vi "configureOutput.vi"(6 "sofwareTrigger?":bool, 8 "error in (no error)":errorcluster, 9 "Data":variant, 10 "Config":T1, 11 "SpinCore in":refnum<class "SpinCore.lvclass">) -> (0 "error out":errorcluster, 3 "SpinCore out":refnum<class "SpinCore.lvclass">)   [LabVIEW 2009, in "Hardware.lvlib" / "Channels.lvlib" / "SpinCore.lvclass"]
doc: "Data is a varient cluster. \n\nThe varient is transformed into the correct cluster, and that cluster is stored.\n(Not Implemented for Ramp function)"
uses:
  SpinCore.lvclass
  Generic/DDSOutput.lvclass
  SpinCore.lvclass/SpinCore.ctl
panel:
  out "Data":dbl
  out "load time":dbl
  out "data (time, freq, amplitude, phase)":dbl[][](array[numeric]) format="%#.7g"
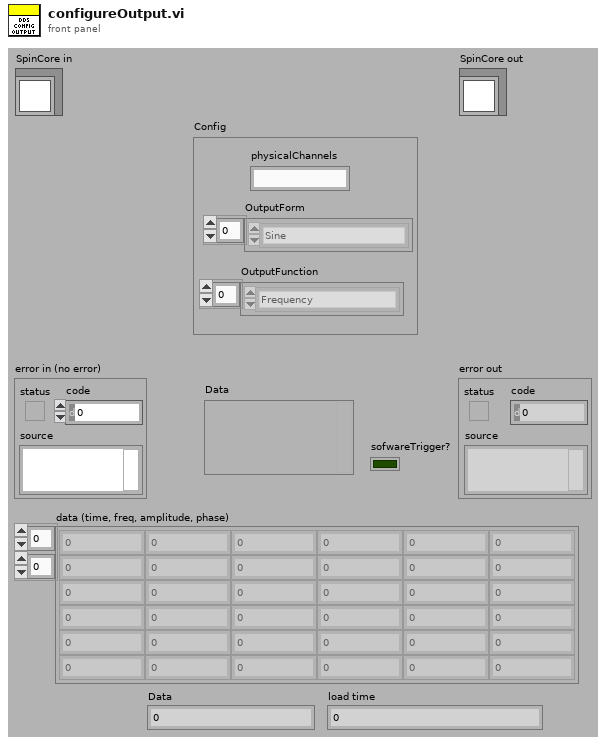
[diagram p1: front panel]
types:
  T1 = cluster{"OutputForm":enum16{"Sine", "Square", "Triangle", "Arbitrary"}[], "OutputFunction":enum16{"Frequency", "Ramp", "Sequence"}[], "physicalChannels":string}
  T2 = cluster{"Frequency(MHz)":dbl, "Amplitude":dbl, "Phase":dbl, "OutputForm":enum16{"Sine", "Square", "Triangle", "Arbitrary"}}[]
  T3 = cluster{"data (time, freq, amplitude, phase)":dbl[][]}
  T4 = cluster{"data (time, freq, amplitude, phase)":dbl[][]}[]
  T5 = cluster{"Frequency(MHz)":dbl, "Amplitude":dbl, "Phase":dbl, "OutputForm":enum16{"Sine", "Square", "Triangle", "Arbitrary"}}
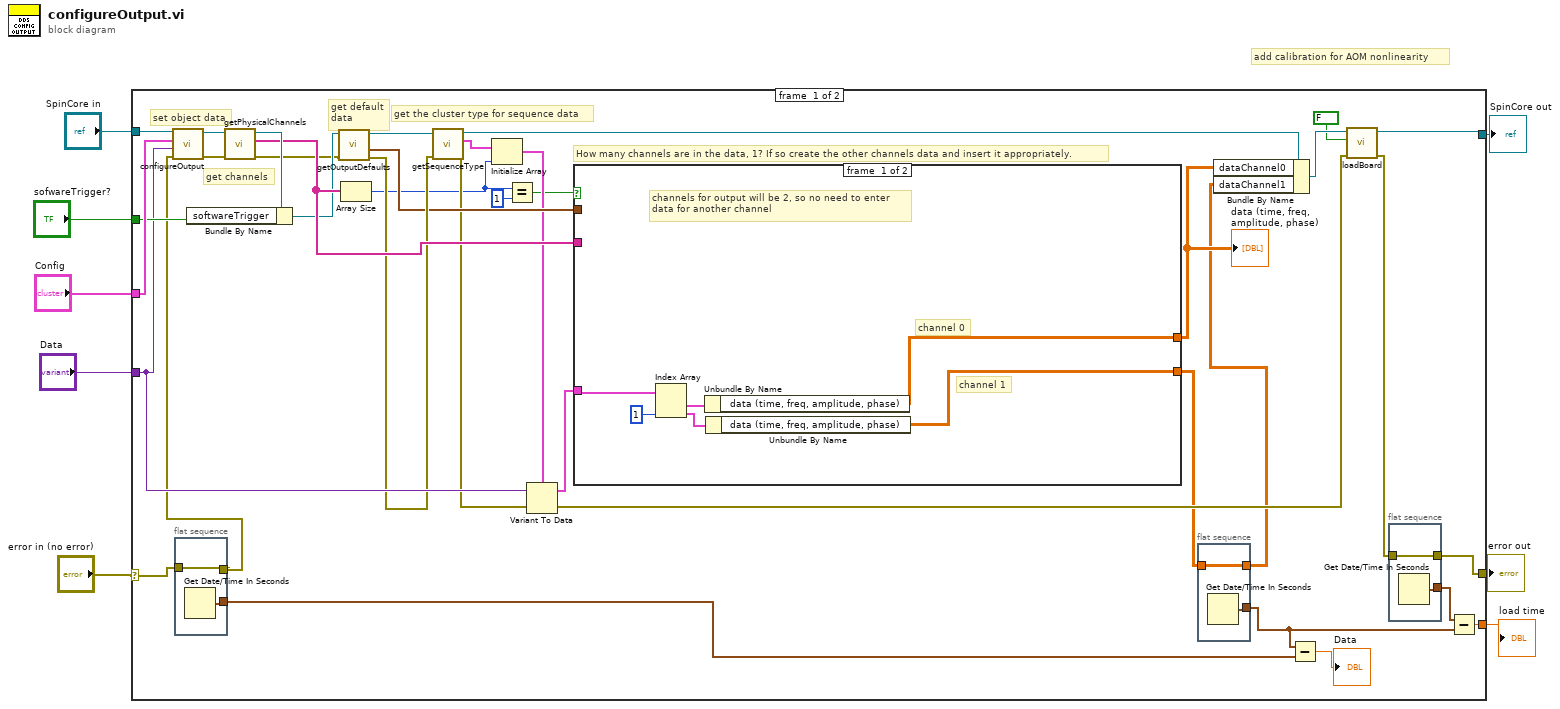
[diagram p0: block diagram]
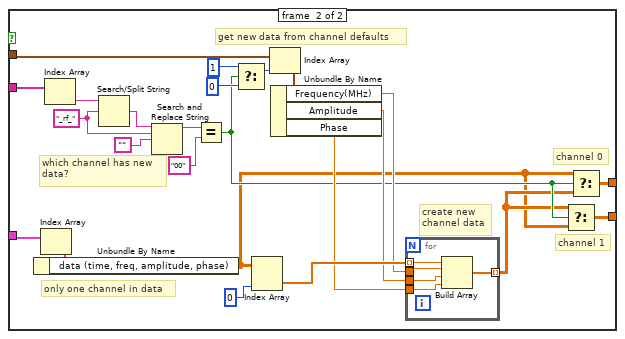
[diagram p2: hidden frame]
diagram:
  # "add calibration for AOM nonlinearity"
  n1 = case shown="No Error" "error in (no error)" {
    selector: "error in (no error)" -> [w16 w87]
    tunnel: [w20 w87] -> w8
    tunnel: [w42 w88] -> w7
    tunnel: "SpinCore in" -> [w45 w88]
    tunnel: "Config" -> [w44 _]
    tunnel: "Data" -> [w36 _]
    tunnel: "sofwareTrigger?" -> [w41 _]
    tunnel: [w17 _] -> w1
    frame #0 {
      # "get default\ndata"
      # "get channels"
      # "set object data"
      # "get the cluster type for sequence data"
      # "How many channels are in the data, 1? If so create the other channels data and insert it appropriately."
      n2 = call-parent "configureOutput.vi"("error in (no error)"=w15, "Data"=w36, "Config"=w44, "DDSOutput in"=w45) -> ("error out"=w40:errorcluster, "DDSOutput out"=w39:refnum<class "SpinCore.lvclass">)  [unwired: 6 in]
      n3 = flat-sequence {
        tunnel: [w47] -> w15
        tunnel: w16 -> [w47]
        tunnel: [w46] -> w10
        frame #0 {
          n4 = Get Date/Time In Seconds() -> (seconds since 1Jan1904=w46:timestamp)
        }
      }
      n5 = call "getPhysicalChannels.vi"("error in (no error)"=w40, "DDSOutput in"=w39) -> ("error out"=w32:errorcluster, "physicalChannels"=w37:string[], "DDSOutput out"=w38:refnum<class "SpinCore.lvclass">)  [unwired: 7 in]
      n6 = Bundle By Name(cluster=w38, "softwareTrigger"=w41) -> (w33:refnum<class "SpinCore.lvclass">)
      n7 = call "getOutputDefaults.vi"("error in (no error)"=w32, "DDSOutput in"=w33) -> ("error out"=w31:errorcluster, "Defaults"=w30:T2, "DDSOutput out"=w34:refnum<class "SpinCore.lvclass">)  [unwired: 6 in, 1 out]
      n8 = Array Size(array=w37) -> (size(s)=w23:i32)
      n9 = call "getSequenceType.vi"("error in (no error)"=w31, "DDSOutput in"=w34) -> ("error out"=w28:errorcluster, "Sequence"=w29:T3, "DDSOutput out"=w26:refnum<class "SpinCore.lvclass">)  [unwired: 7 in]
      n10 = Initialize Array(w29, w23) -> (w27:T4)
      n11 = Equal?(x=w23, y=1) -> (x = y?=w22:bool)
      n12 = Variant To Data(error in=w28, Variant=w36, type=w27) -> (error out=w14:errorcluster, data=w25:T4)
      n13 = case shown="True" w22 {
        tunnel: w37 -> [_ w77]
        tunnel: w30 -> [_ w70]
        tunnel: w25 -> [w57 w71]
        tunnel: [w55 w61] -> w24
        tunnel: [w53 w60] -> w13
        frame #0 {
          # "channel 1"
          # "channel 0"
          # "channels for output will be 2, so no need to enter\ndata for another channel"
          n14 = Index Array(array=w57, index #2=1) -> (element #1=w56:T3, element #2=w54:T3)  [unwired: 1 in]
          n15 = Unbundle By Name(w56) -> ("data (time, freq, amplitude, phase)"=w55:dbl[][])
          n16 = Unbundle By Name(w54) -> ("data (time, freq, amplitude, phase)"=w53:dbl[][])
        }
        frame #1 {
          w79 = "_rf_"
          # "get new data from channel defaults"
          # "only one channel in data"
          # "create new\nchannel data"
          # "channel 1"
          # "channel 0"
          # "which channel has new\ndata?"
          n17 = Index Array(array=w71) -> (element=w69:T3)  [unwired: 1 in]
          n18 = Unbundle By Name(w69) -> ("data (time, freq, amplitude, phase)"=w58:dbl[][])
          n19 = Index Array(array=w77) -> (element=w81:string)  [unwired: 1 in]
          n20 = Search/Split String(string=w81, search string/char (-)=w79) -> (match + rest of string=w80:string)  [unwired: 1 in, 2 out]
          n21 = Search and Replace String(input string=w80, search string=w79, replace string="") -> (result string=w75:string)  [unwired: 5 in, 3 out]
          n22 = Equal?(x=w75, y="00") -> (x = y?=w62:bool)
          n23 = Select(t=1, s=w62, f=0) -> (s? t:f=w74:i32)
          n24 = Index Array(array=w58, index (col)=0) -> (element=w66:dbl[])  [unwired: 1 in]
          n25 = Index Array(array=w70, index=w74) -> (element=w68:T5)
          n26 = Unbundle By Name(w68) -> ("Frequency(MHz)"=w65:dbl, "Amplitude"=w64:dbl, "Phase"=w63:dbl)
          n27 = for {
            tunnel: w66 -> [w86] mode=indexing
            tunnel: w65 -> [w85]
            tunnel: w64 -> [w84]
            tunnel: w63 -> [w83]
            tunnel: [w82] -> w59 mode=indexing
            n28 = Build Array(w86, w85, w84, w83) -> (w82:dbl[])
          }
          n29 = Select(t=w59, s=w62, f=w58) -> (s? t:f=w60:dbl[][])
          n30 = Select(t=w58, s=w62, f=w59) -> (s? t:f=w61:dbl[][])
        }
      }
      "data (time, freq, amplitude, phase)" <- w24
      n31 = flat-sequence {
        tunnel: [w51] -> w11
        tunnel: [w50] -> w12
        tunnel: w13 -> [w50]
        frame #0 {
          n32 = Get Date/Time In Seconds() -> (seconds since 1Jan1904=w51:timestamp)
        }
      }
      n33 = Bundle By Name(cluster=w26, "dataChannel0"=w24, "dataChannel1"=w12) -> (w43:refnum<class "SpinCore.lvclass">)
      n34 = Subtract(x=w11, y=w10) -> (x-y=→"Data":dbl)
      n35 = call "loadBoard.vi"("error in (no error)"=w14, "continuous"=FALSE, "SpinCore in"=w43) -> ("error out"=w19:errorcluster, "SpinCore out"=w42:refnum<class "SpinCore.lvclass">)  [unwired: 7 in]
      n36 = flat-sequence {
        tunnel: [w49] -> w18
        tunnel: [w48] -> w20
        tunnel: w19 -> [w48]
        frame #0 {
          n37 = Get Date/Time In Seconds() -> (seconds since 1Jan1904=w49:timestamp)
        }
      }
      n38 = Subtract(x=w18, y=w11) -> (x-y=w17:dbl)
    }
    frame #1 {
    }
  }
  "error out" <- w8
  "SpinCore out" <- w7
  "load time" <- w1
